vi "RS_SMBV100A_ImportToNMEA.vi"(8 "error in":errorcluster, 11 "Dynam waypoints":T1 {"Time" format="%<%.3X>T"; "Speed" format="%#.10g"; "Heigth" format="%#.10g"; "Longitude" format="%#.10g"; "Latitude" format="%#.10g"}) -> (0 "error out":errorcluster)   [LabVIEW 2018]
uses:
  RS_SMBV100A_DynamWaypoints.ctl
  RS_SMBV100A_DynamWaypoint.ctl
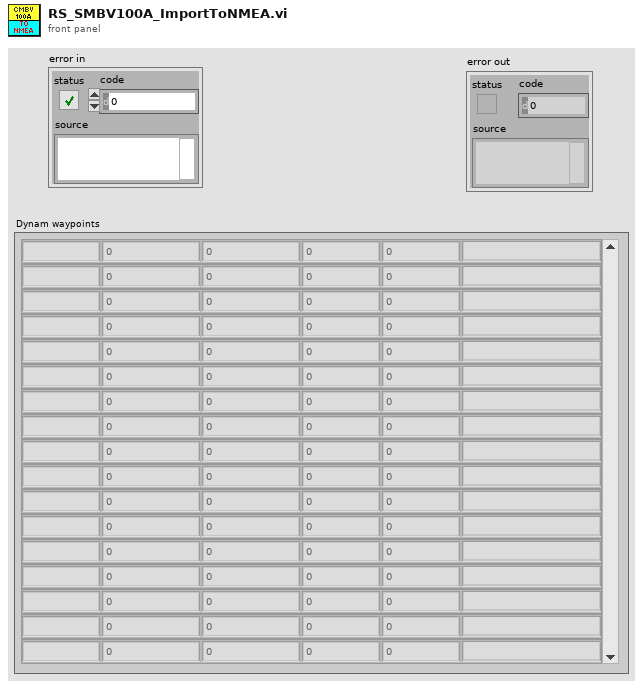
[diagram p1: front panel]
types:
  T1 = typedef "RS_SMBV100A_DynamWaypoints.ctl" = T2[]
  T2 = typedef "RS_SMBV100A_DynamWaypoint.ctl" = cluster{"Time":timestamp, "Latitude":ext, "Longitude":ext, "Heigth":dbl, "Speed":dbl, "Scenario":string}
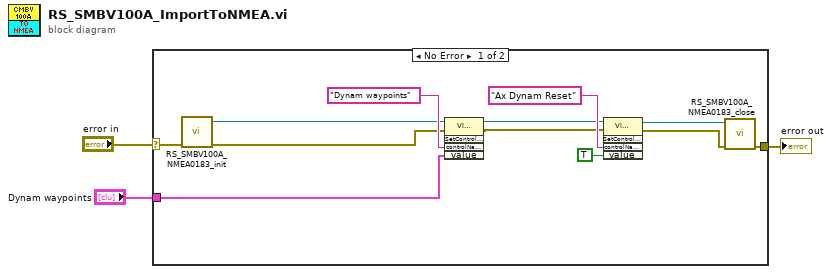
[diagram p0: block diagram]
diagram:
  n1 = case shown="No Error" "error in" {
    selector: "error in" -> [w7 w16]
    tunnel: [w8 w16] -> w3
    tunnel: "Dynam waypoints" -> [w4 _]
    frame No Error {
      n2 = call "RS_SMBV100A_NMEA0183_init.vi"("error in"=w7) -> ("error out"=w13:errorcluster, "NMEA0183 Ref"=w14:refnum<k7>)  [unwired: 9 in]
      n3 = invoke class="VirtualInstrument" method="SetControlValue"(reference=w14, error in=w13, "controlName"="Dynam waypoints", "value"=w4) -> (reference out=w6:refnum<k7>, error out=w5:errorcluster)  [unwired: 1 in, 3 out]
      n4 = invoke class="VirtualInstrument" method="SetControlValue"(reference=w6, error in=w5, "controlName"="Ax Dynam Reset", "value"=TRUE ("Threshold Data.Dark Characters")) -> (reference out=w9:refnum<k7>, error out=w10:errorcluster)  [unwired: 1 in, 3 out]
      n5 = call "RS_SMBV100A_NMEA0183_close.vi"("error in"=w10, "NMEA0183 Ref"=w9) -> ("error out"=w8:errorcluster)  [unwired: 8 in]
    }
    frame Error {
    }
  }
  "error out" <- w3
